vi "Main_LTC1859.vi"() -> ()   [LabVIEW 2015]
uses:
  <vilib>/myRIO/Instrument Drivers/Onboard IO/SPI/typedefs/SPI User Configuration.ctl
  <vilib>/myRIO/Common/Instrument Driver Framework/myRIO v1.0/SPI/typedefs/SPI Clock Phase.ctl
  <vilib>/myRIO/Common/Instrument Driver Framework/myRIO v1.0/SPI/typedefs/SPI Clock Polarity.ctl
  <vilib>/myRIO/Common/Instrument Driver Framework/myRIO v1.0/SPI/typedefs/SPI Data Direction.ctl
  <vilib>/myRIO/Common/Instrument Driver Framework/myRIO v1.0/SPI/typedefs/SPI Frame Length.ctl
  <vilib>/myRIO/Instrument Drivers/Onboard IO/SPI/typedefs/SPI Reference.ctl
  <vilib>/myRIO/Common/Instrument Driver Framework/Utilities/typedefs/myRIO Generic Hardware Reference.ctl
  <vilib>/myRIO/Common/Instrument Driver Framework/Utilities/typedefs/Hardware Version Enum.ctl
  <vilib>/myRIO/Common/Instrument Driver Framework/Utilities/typedefs/myRIO v1.0 Reference.ctl
  <vilib>/myRIO/Common/Instrument Driver Framework/Utilities/typedefs/Generic FPGA Reference.ctl
  <vilib>/myRIO/Common/Instrument Driver Framework/myRIO v1.0/SPI/typedefs/SPI Channels Enum.ctl
  <vilib>/myRIO/Instrument Drivers/Onboard IO/SPI/typedefs/SPI Configuration.ctl
  <vilib>/userdefined/High Color/nirio_resource_hc.ctl
  <vilib>/myRIO/Common/Instrument Driver Framework/Utilities/vis/Is FPGA Ref Available.vi
  <vilib>/myRIO/Common/Instrument Driver Framework/myRIO v1.0/SPI/vis/myRIO v1.1 Open SPI.vi
  <vilib>/myRIO/Instrument Drivers/Onboard IO/SPI/vis/Configure.vi
  <vilib>/myRIO/Instrument Drivers/Onboard IO/SPI/vis/Write.vi
  <vilib>/myRIO/Instrument Drivers/Onboard IO/SPI/vis/Read.vi
  <vilib>/myRIO/Instrument Drivers/Onboard IO/DIO/vis/Write.vi
  <vilib>/myRIO/Common/Instrument Driver Framework/Utilities/vis/Validate Channels.vi
  <vilib>/myRIO/Common/Instrument Driver Framework/myRIO v1.0/SPI/vis/myRIO v1.0 Reserve SPI.vi
  <vilib>/myRIO/Instrument Drivers/Onboard IO/SPI/vis/Write Read.vi
  <vilib>/myRIO/Common/Instrument Driver Framework/myRIO v1.0/SPI/vis/myRIO v1.0 Build MUX Configuration SPI.vi
  <vilib>/myRIO/Common/Instrument Driver Framework/myRIO v1.0/Resource Manager/vis/myRIO v1.0 Reserve Channel List.vi
  <vilib>/myRIO/Common/Instrument Driver Framework/myRIO v1.0/Resource Manager/vis/myRIO v1.0 Create Configuration List.vi
  <vilib>/myRIO/Common/Instrument Driver Framework/myRIO v1.0/Resource Manager/vis/myRIO v1.0 Reserve Channel.vi
  <vilib>/myRIO/Common/Instrument Driver Framework/myRIO v1.0/Resource Manager/vis/myRIO v1.0 Unreserve Channel.vi
  <vilib>/myRIO/Common/Instrument Driver Framework/myRIO v1.0/Resource Manager/vis/myRIO v1.0 Build Mutex Name.vi
  <vilib>/myRIO/Instrument Drivers/Onboard IO/DIO/vis/Smart Open.vi
  <vilib>/Utility/error.llb/Error Cluster From Error Code.vi
  <vilib>/myRIO/Common/Instrument Driver Framework/myRIO v1.0/DIO/vis/myRIO v1.0 Write DIO.vi
  <vilib>/Utility/VariantDataType/GetNumericInfo.vi
  <vilib>/myRIO/Common/Instrument Driver Framework/myRIO v1.0/myRIO v1.1 Open.vi
  <vilib>/myRIO/Common/Instrument Driver Framework/Utilities/vis/IO Manager.vi
  <vilib>/myRIO/Common/Instrument Driver Framework/Utilities/vis/Configuration Manager.vi
  <vilib>/myRIO/Common/Instrument Driver Framework/myRIO v1.0/Resource Manager/vis/myRIO v1.0 Configure IO.vi
  <vilib>/myRIO/Common/Instrument Driver Framework/myRIO v1.0/myRIO v1.0 Close.vi
  <vilib>/myRIO/Common/Instrument Driver Framework/myRIO v1.0/SPI/vis/myRIO v1.0 Configure SPI.vi
  <vilib>/myRIO/Common/Instrument Driver Framework/myRIO v1.0/SPI/vis/myRIO v1.0 Write Read SPI.vi
  <vilib>/myRIO/Express VI/Onboard IO/SPI/SPI Express VI.xnode
  <vilib>/myRIO/Instrument Drivers/Onboard IO/SPI/vis/myRIO SPI Open.xnode
  <vilib>/myRIO/Instrument Drivers/Onboard IO/SPI/SPI.lvlib
panel:
  in  "chhose your measurement mode":enum32{"Single", "Differential"}(tab)
  in  "Channel":dbl min=0.0 max=7.0
  in  "Pair":dbl min=0.0 max=3.0
  out "Voltage":dbl(graph)
  in  "?":bool
  # "choose\n0 for 0 and 1\n1 for 2 and 3\n2 for 4 and 5\n3 for 6 and 7"
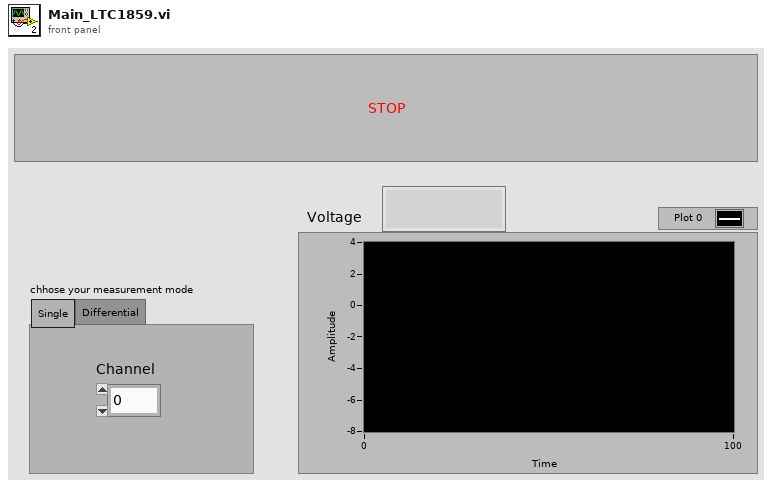
[diagram p1: front panel]
types:
  T1 = typedef "SPI.lvlib/SPI Reference.ctl" = cluster{"myRIO Reference":T2, "SPI Channels Enum":T6, "SPI Configuration":T7}
  T2 = typedef "myRIO Generic Hardware Reference.ctl" = cluster{"myRIO Model":T3, "myRIO Hardware Reference":T4}
  T3 = typedef "Hardware Version Enum.ctl" = enum16{"Unknown", "myRIO-1900", "myRIO-1950", "roboRIO"}
  T4 = typedef "myRIO v1.0 Reference.ctl" = cluster{"Generic FPGA Reference":T5, "Allow multiple opens":bool}
  T5 = typedef "Generic FPGA Reference.ctl" = refnum<k20>
  T6 = typedef "SPI Channels Enum.ctl" = enum16{"Not Connected", "A/SPI", "B/SPI", "SPI/SPI"}
  T7 = typedef "SPI.lvlib/SPI Configuration.ctl" = cluster{"Frequency [Hz]":dbl, "Clock Phase":T8, "Clock Polarity":T9, "Data Direction":T10, "Frame Length":T11}
  T8 = typedef "SPI Clock Phase.ctl" = enum8{"Leading", "Trailing"}
  T9 = typedef "SPI Clock Polarity.ctl" = enum8{"Low", "High"}
  T10 = typedef "SPI Data Direction.ctl" = enum8{"Most significant bit first", "Least significant bit first"}
  T11 = typedef "SPI Frame Length.ctl" = u8
  T12 = typedef "SPI.lvlib/SPI User Configuration.ctl" = cluster{"Frequency [Hz]":dbl, "Clock Phase":T8, "Clock Polarity":T9, "Data Direction":T10, "Frame Length":T11}
  T13 = typedef "nirio_resource_hc.ctl" = tag
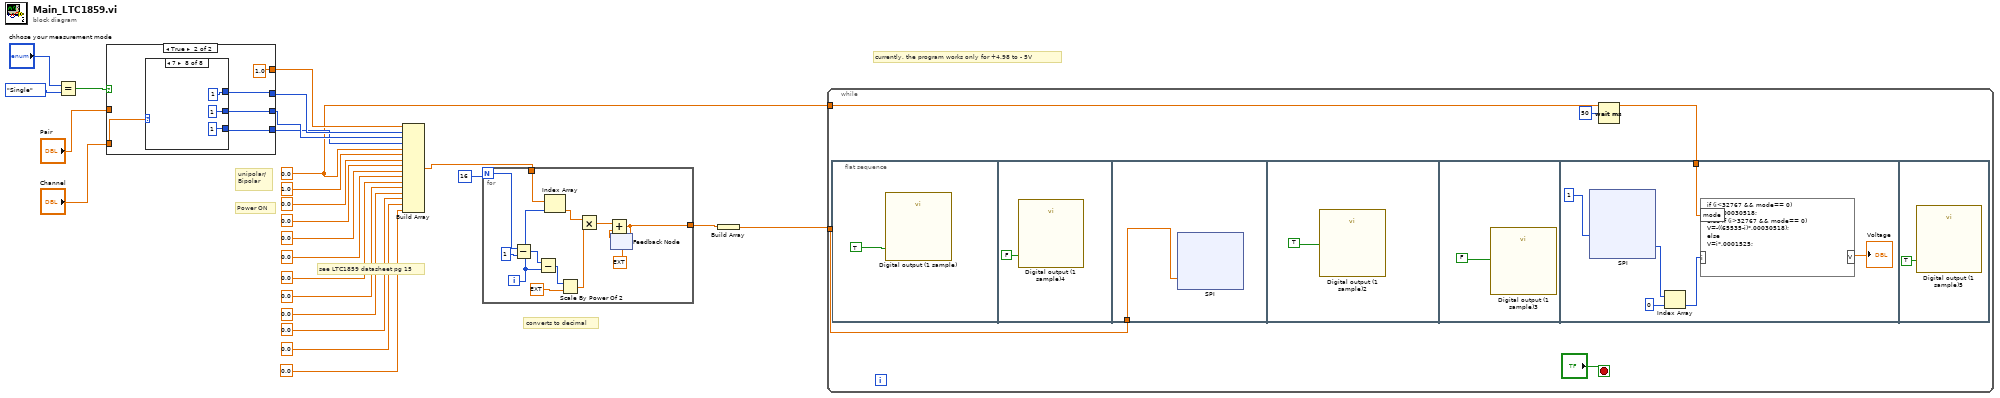
[diagram p0: block diagram]
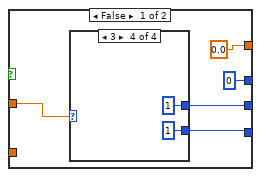
[diagram p2: hidden frame]
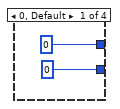
[diagram p3: hidden frame]
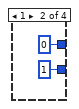
[diagram p4: hidden frame]
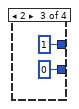
[diagram p5: hidden frame]
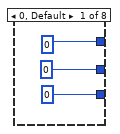
[diagram p6: hidden frame]
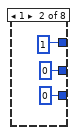
[diagram p7: hidden frame]
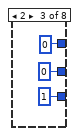
[diagram p8: hidden frame]
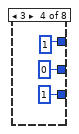
[diagram p9: hidden frame]
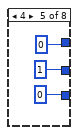
[diagram p10: hidden frame]
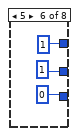
[diagram p11: hidden frame]
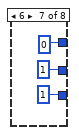
[diagram p12: hidden frame]
diagram:
  w4 = 0.0 ("element")
  # "converts to decimal"
  # "see LTC1859 datasheet pg 15"
  # "Power ON"
  # "unipolar/\nBipolar"
  # "currently, the program works only for +4.98 to - 5V"
  n1 = Equal?(x="chhose your measurement mode", y=enum32{"Single", "Differential"}."Single") -> (x = y?=w1:bool)
  n2 = case shown="True" w1 {
    tunnel: [0.0 ("element") 1.0 ("element")] -> w5
    tunnel: "Pair" -> [w29 _]
    tunnel: "Channel" -> [_ w42]
    tunnel: [0 w41] -> w18
    tunnel: [w27 w40] -> w17
    tunnel: [w26 w39] -> w16
    frame False {
      n3 = case shown="3" w29 {
        tunnel: [0 0 1 1] -> w27
        tunnel: [0 1 0 1] -> w26
        frame 0, Default {
        }
        frame 1 {
        }
        frame 2 {
        }
        frame 3 {
        }
      }
    }
    frame True {
      n4 = case shown="7" w42 {
        tunnel: [0 0 0 0 1 1 1 1] -> w40
        tunnel: [0 0 1 1 0 0 1 1] -> w39
        tunnel: [0 1 0 1 0 1 0 1] -> w41
        frame 0, Default {
        }
        frame 1 {
        }
        frame 2 {
        }
        frame 3 {
        }
        frame 4 {
        }
        frame 5 {
        }
        frame 6 {
        }
        frame 7 {
        }
      }
    }
  }
  n5 = Build Array(w5, w18, w17, w16, w4, 1.0 ("element"), 0.0 ("element"), 0.0 ("element"), 0.0 ("element"), 0.0 ("element"), 0.0 ("element"), 0.0 ("element"), 0.0 ("element"), 0.0 ("element"), 0.0 ("element"), 0.0 ("element")) -> (w8:dbl[])
  n6 = for {
    N: 16 -> [w72]
    tunnel: w8 -> [w80]
    tunnel: [w70] -> w6
    i -> [w75]
    n7 = Subtract(x=w72, y=1) -> (x-y=w73:i32)
    n8 = Subtract(x=w73, y=w75) -> (x-y=w74:i32)
    n9 = Index Array(array=w80, index=w75) -> (element=w69:dbl)
    n10 = Scale By Power Of 2(n=w74, x=ext 1.0) -> (x*2^n=w79:ext)
    n11 = Multiply(x=w69, y=w79) -> (x*y=w78:ext)
    n12 = feedback #1(ext 0.0) -> (w77:ext)
    n13 = Add(x=w78, y=w77) -> (x+y=w70:ext)
    n14 = feedback-in #1(w70) -> ()
  }
  n15 = Build Array(w6) -> (w7:ext[])
  n16 = while {
    tunnel: w7 -> [w82]
    tunnel: w4 -> [w81]
    stop <- "?" stop-if-true
    n17 = flat-sequence {
      tunnel: w82 -> [w87]
      tunnel: w81 -> [w127]
      frame #0 {
        n18 = call "Digital output (1 sample)"("A/DIO0 (Pin 11)"=TRUE) -> ()  [unwired: 26 in, 1 out]
      }
      frame #1 {
        n19 = call "Digital output (1 sample)4"("A/DIO0 (Pin 11)"=FALSE) -> ()  [unwired: 26 in, 1 out]
      }
      frame #2 {
        n20 = xnode "SPI"("Frames to Write"=w87) -> ()  [unwired: 1 in, 1 out]
      }
      frame #3 {
        n21 = call "Digital output (1 sample)2"("A/DIO0 (Pin 11)"=TRUE) -> ()  [unwired: 26 in, 1 out]
      }
      frame #4 {
        n22 = call "Digital output (1 sample)3"("A/DIO0 (Pin 11)"=FALSE) -> ()  [unwired: 26 in, 1 out]
      }
      frame #5 {
        n23 = xnode "SPI "("Frame Count"=u32 1) -> ("Frames Read"=w131:u16[])  [unwired: 1 in, 1 out]
        n24 = Index Array(array=w131, index=0) -> (element=w129:u16)
        n25 = formula code="if (i<32767 && mode== 0)\nV=i*.00030518;\nelse if (i>32767 && mode== 0)\nV=-((65535-i)*.00030518);\nelse\nV=i*.0001525;"("i"=w129, "mode"=w127) -> ("V"=→"Voltage":dbl)
      }
      frame #6 {
        n26 = call "Digital output (1 sample)5"("A/DIO0 (Pin 11)"=TRUE) -> ()  [unwired: 26 in, 1 out]
      }
    }
    n27 = Wait (ms)(milliseconds to wait=u32 50) -> ()  [unwired: 1 out]
  }
